vi "Stoermeldungen abarbeiten.vi"(0 "Störungen 129-192":u64, 1 "Störungen 193-256":u64, 2 "Störungen 257-320":u64, 3 "Störungen 321-384":u64, 4 "Störungen 385-448":u64, 5 "Störungen 449-512":u64, 7 "Fehler (Eingang)":errorcluster caption="Fehler (Eingang, kein Fehler)") -> (27 "Fehler (Ausgang)":errorcluster)   [LabVIEW 2020, in "Stoerungen.lvlib"]
uses:
  Stoerungen.lvlib
  FGV Stoerung aufnehmen Aktion.ctl
  Allgemein/Aktion FGV Aufheizphase.ctl
  Seiten/Anlagengrenzwerte/FGV Anlagengrenzwerte Aktionen.ctl
  cRIO/PC/Kommunikation mit cRIO.lvlib
  Allgemein/allgemeine Sub-VIs.lvlib
  Seiten/Anlagengrenzwerte/Anlagengrenzwerte.lvlib
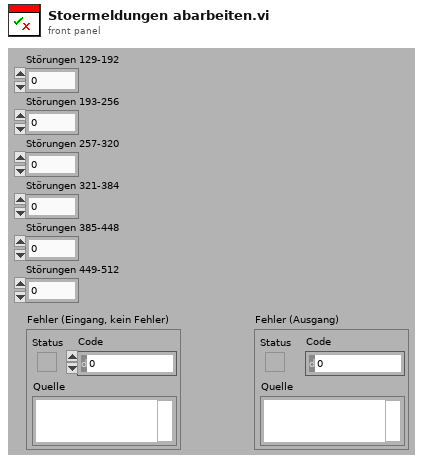
[diagram p1: front panel]
types:
  T1 = typedef "allgemeine Sub-VIs.lvlib/Aktion FGV Aufheizphase.ctl" = enum16{"init", "lesen", "PNS Filterblock", "PNS HL1", "PNS HL2", "PNS HL3", "PNS HL4", "FTIR Messzelle", "HL 1", "HL 2", "HL zu FTIR", "auswerten"}
  T2 = typedef "Anlagengrenzwerte.lvlib/FGV Anlagengrenzwerte Aktionen.ctl" = enum16{"Lesen", "Grenzwerte schreiben"}
  T3 = typedef "Stoerungen.lvlib/FGV Stoerung aufnehmen Aktion.ctl" = enum16{"Initialisieren", "Schreiben", "Lesen", "Quittieren", "quit. löschen"}
  T4 = typedef "Anlagengrenzwerte.lvlib/Anlagen-Grenzwerte Anzeige.ctl" = cluster{"Eingangsdruck FT-IR:":T5, "Durchfluss FT-IR:":T5, "Durchfluss CalGas:":T5, "Druck Ausgang:":T5, "Druck Kalter Block:":T5, "Heizleitungen intern:":T5, "Heizleitung zu FT-IR:":T5, "Heizung Filterblock:":T5, "Heizung Pumpe:":T5, "Heizleitung Extern SP1:":T5, "Heizleitung Extern SP2:":T5, "FT-IR Heizung Messzelle:":T5, "Schaltschranktemperatur:":T5, "Gaskühler:":T5}
  T5 = typedef "Anlagengrenzwerte.lvlib/Anlagen-Parameter Anzeige.ctl" = cluster{"Sollwert":sgl, "Warn-Min":sgl, "Warn-Max":sgl, "Abschalt-Min":sgl, "Abschalt-Max":sgl, "Regler":u16}
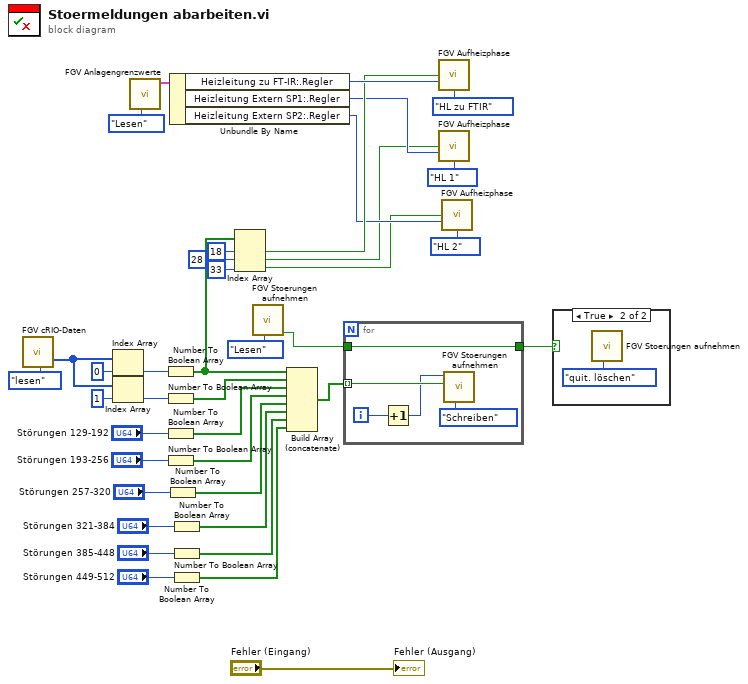
[diagram p0: block diagram]
diagram:
  n1 = call "FGV cRIO-Daten.vi"("Aktion"=enum16{"lesen", "schreiben"}."lesen") -> ("Störungen"=w30:u64[])  [unwired: 9 in, 9 out]
  n2 = Index Array(array=w30, index=0 ("Index")) -> (element=w27:u64)
  n3 = Index Array(array=w30, index=1 ("Index")) -> (element=w26:u64)
  n4 = call "FGV Anlagengrenzwerte.vi"("Aktion"=FGV_Anlagengrenzwerte_Aktionen."Lesen") -> ("Anlagen-Grenzwerte Anzeige"=w9:T4)  [unwired: 10 in]
  n5 = Number To Boolean Array(number=w27) -> (Boolean array=w15:bool[])
  n6 = Number To Boolean Array(number=w26) -> (Boolean array=w36:bool[])
  n7 = Number To Boolean Array(number="Störungen 129-192") -> (Boolean array=w37:bool[])
  n8 = Number To Boolean Array(number="Störungen 193-256") -> (Boolean array=w38:bool[])
  n9 = Number To Boolean Array(number="Störungen 257-320") -> (Boolean array=w19:bool[])
  n10 = Unbundle By Name(w9) -> ("Heizleitung zu FT-IR:.Regler"=w8:u16, "Heizleitung Extern SP1:.Regler"=w5:u16, "Heizleitung Extern SP2:.Regler"=w3:u16)
  n11 = Number To Boolean Array(number="Störungen 321-384") -> (Boolean array=w18:bool[])
  n12 = Number To Boolean Array(number="Störungen 385-448") -> (Boolean array=w17:bool[])
  n13 = Number To Boolean Array(number="Störungen 449-512") -> (Boolean array=w16:bool[])
  n14 = Index Array(array=w15, index #1=18 ("Index"), index #2=28 ("Index"), index #3=33 ("Index")) -> (element #1=w7:bool, element #2=w2:bool, element #3=w1:bool)
  n15 = call "FGV Stoerungen aufnehmen.vi"("FGV Störung aufnehmen Aktion"=FGV_Stoerung_aufnehmen_Aktion."Lesen") -> ("quittieren?"=w34:bool)  [unwired: 7 in, 3 out]
  n16 = Build Array (concatenate)(w15, w36, w37, w38, w19, w18, w17, w16) -> (w39:bool[])
  n17 = for {
    tunnel: w39 -> [w44] mode=indexing
    tunnel: w34 -> [w40]
    tunnel: [w40] -> w35
    i -> [w42]
    n18 = Increment(x=w42) -> (x+1=w41:i32)
    n19 = call "FGV Stoerungen aufnehmen.vi"("FGV Störung aufnehmen Aktion"=FGV_Stoerung_aufnehmen_Aktion."Schreiben", "Störung ein"=w44, "Meldungs-Nummer"=w41) -> ()  [unwired: 5 in, 4 out]
  }
  n20 = call "FGV Aufheizphase.vi"("Error"=w7, "Aktiv/Inaktiv"=w8, "Aktion"=Aktion_FGV_Aufheizphase."HL zu FTIR") -> ()  [unwired: 10 in, 3 out]
  n21 = call "FGV Aufheizphase.vi"("Error"=w2, "Aktiv/Inaktiv"=w5, "Aktion"=Aktion_FGV_Aufheizphase."HL 1") -> ()  [unwired: 10 in, 3 out]
  n22 = call "FGV Aufheizphase.vi"("Error"=w1, "Aktiv/Inaktiv"=w3, "Aktion"=Aktion_FGV_Aufheizphase."HL 2") -> ()  [unwired: 10 in, 3 out]
  n23 = case shown="True" w35 {
    frame False {
    }
    frame True {
      n24 = call "FGV Stoerungen aufnehmen.vi"("FGV Störung aufnehmen Aktion"=FGV_Stoerung_aufnehmen_Aktion."quit. löschen") -> ()  [unwired: 7 in, 4 out]
    }
  }
  "Fehler (Ausgang)" <- "Fehler (Eingang)"
